vi "Clean-up.vi"(8 "error in (no error)":errorcluster, 11 "File in":refnum<class "File.lvclass">) -> (0 "error out":errorcluster, 3 "File out":refnum<class "File.lvclass">)   [LabVIEW 2016, in "File.lvclass"]
uses:
  File.lvclass
  File.lvclass/File.ctl
  Write tdms stream.vi
  Read Is open.vi
  Read tdms stream.vi
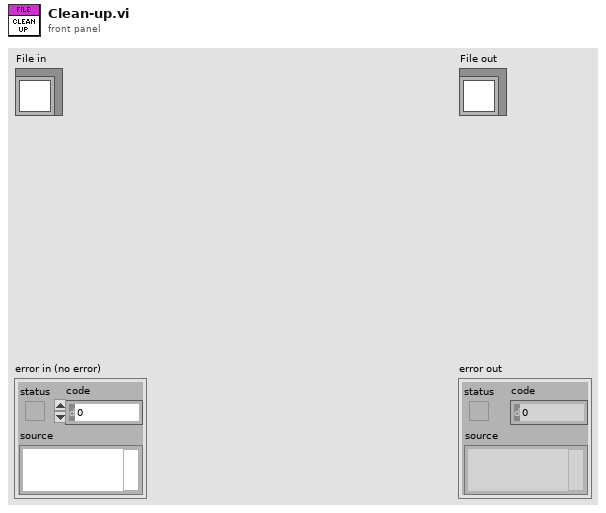
[diagram p1: front panel]
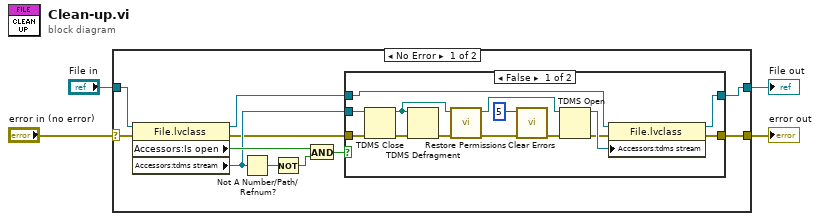
[diagram p0: block diagram]
diagram:
  n1 = case shown="No Error" "error in (no error)" {
    selector: "error in (no error)" -> [w6 w33]
    tunnel: [w5 w33] -> w3
    tunnel: [w7 w32] -> w1
    tunnel: "File in" -> [w12 w32]
    frame No Error {
      n2 = property class="File.lvclass"(reference=w12, error in=w6) -> (reference out=w8:refnum<class "File.lvclass">, error out=w10:errorcluster, "Accessors:Is open"=w13:bool, "Accessors:tdms stream"=w11:refnum<k34>)
      n3 = Not A Number/Path/Refnum?(number/path/refnum=w11) -> (NaN/Path/Refnum?=w14:bool)
      n4 = Not(x=w14) -> (.not. x?=w15:bool)
      n5 = And(x=w13, y=w15) -> (x .and. y?=w9:bool)
      n6 = case shown="False" w9 {
        tunnel: w11 -> [w29 _]
        tunnel: w10 -> [w28 w31]
        tunnel: w8 -> [w25 w30]
        tunnel: [w22 w30] -> w7
        tunnel: [w21 w31] -> w5
        frame False {
          n7 = TDMS Close(8:w28, 11:w29) -> (0:w27:errorcluster, 3:w16:path)
          n8 = TDMS Defragment(4:w27, 7:w16) -> (0:w26:errorcluster)
          n9 = call "Restore Permissions.vi"("Error In"=w26, "File Path"=w16) -> ("Error Out"=w18:errorcluster, "Duplicate File Path"=w17:path)  [unwired: 6 in, 2 out]
          n10 = call <vilib>:"Clear Errors.vi"("error in (no error)"=w18, "specific error code to clear (0: all)"=5) -> ("error out"=w20:errorcluster)  [unwired: 4 in, 1 out]
          n11 = TDMS Open(8:w20, 11:w17) -> (0:w23:errorcluster, 3:w24:refnum<k34>)  [unwired: 5 in]
          n12 = property class="File.lvclass"(reference=w25, error in=w23, "Accessors:tdms stream"=w24) -> (reference out=w22:refnum<class "File.lvclass">, error out=w21:errorcluster)
        }
        frame True {
        }
      }
    }
    frame Error {
    }
  }
  "error out" <- w3
  "File out" <- w1
